vi "Dashboard Main.vi"() -> ()   [LabVIEW 2017]
uses:
  <vilib>/Rock Robotics/Network Tables/NT Read Numeric Array.vi
  <vilib>/Rock Robotics/Network Tables/NT Read Number.vi
  <vilib>/Rock Robotics/Network Tables/NT Write Numeric Array.vi
panel:
  out "Camera Info":cluster{"Mbps LED":bool, "Mbps":dbl, "fps":dbl} {"fps" format="%#.1g"; "Mbps" format="%#.1g"}
  in  "Camera Settings":T1={"Frame Rate"=30, "Compression"=30, "Size"=1, "DB Camera Config"=FALSE} {"Frame Rate" scale=1.0..30.0; "Compression" scale=100.0..-1.0; "Size" items=["640x480", "320x240", "160x120"]}
  in  "TCP":refnum<k5>
  out "Robot IP":string
  in  "Dashboard Tab":T2(tab)
  in  "Select Auto":string(combo)="Select Autonomous ..."
  out "NT Connection":bool
  out "MotorChart R":cluster{"Numeric":dbl, "Numeric":dbl}(graph)
  out "MotorChart L":cluster{"Numeric":dbl, "Numeric":dbl}(graph)
  out "MotorSliders R":cluster{"MotorSlide1":dbl, "MotorSlide2":dbl} {"MotorSlide2" scale=-1.0..1.0 scale format="%#_2e"; "MotorSlide1" scale=-1.0..1.0 scale format="%#_2e"}
  out "MotorSliders L":cluster{"MotorSlide1":dbl, "MotorSlide2":dbl} {"MotorSlide2" scale=-1.0..1.0 scale format="%#_2e"; "MotorSlide1" scale=-1.0..1.0 scale format="%#_2e"}
  out "JS1 Z":dbl(slide) scale=-1.0..1.0 scale format="%#_2e"
  out "JS1 Graph":cluster{"X":dbl, "Y":dbl}[](graph)
  out "JS1 Buttons":T3
  out "JS2 Z":dbl(slide) scale=-1.0..1.0 scale format="%#_2e"
  out "JS2 Graph":cluster{"X":dbl, "Y":dbl}[](graph)
  out "JS2 Buttons":T3
  out "Mode":T4(ring)=enum."Auto Disabled"
  out "Encoder Graph":dbl[][](graph)
  out "JS1 Graph 2":cluster{"X":dbl, "Y":dbl}[](graph)
  out "JS1 Z 2":dbl(slide) scale=-1.0..1.0 scale format="%#_2e"
  out "Waveform Graph":dbl[][](graph)
  in  "P-Value":dbl(slide) scale=-2.0..2.0
  in  "I-Value":dbl(slide) scale=-2.0..2.0
  in  "D-Value":dbl(slide) scale=-2.0..2.0
  in  "H-Lower":dbl(slide) scale=0.0..179.0
  in  "V-Lower":dbl(slide) scale=0.0..255.0
  in  "S-Lower":dbl(slide) scale=0.0..255.0
  in  "S-Higher":dbl(slide) scale=0.0..255.0
  in  "V-Higher":dbl(slide) scale=0.0..255.0
  in  "H-Upper":dbl(slide) scale=0.0..179.0
  out "Tree":string(tree)
  out "Camera Image":T5(plugin-control)
  out "Background":bool
  in  "Camera Name":string(combo)="No Camera Selection"
  # "HW"
  # "Joysticks"
  # "Drive Motors"
  # "Front"
  # "Right"
  # "Left"
  # "Back"
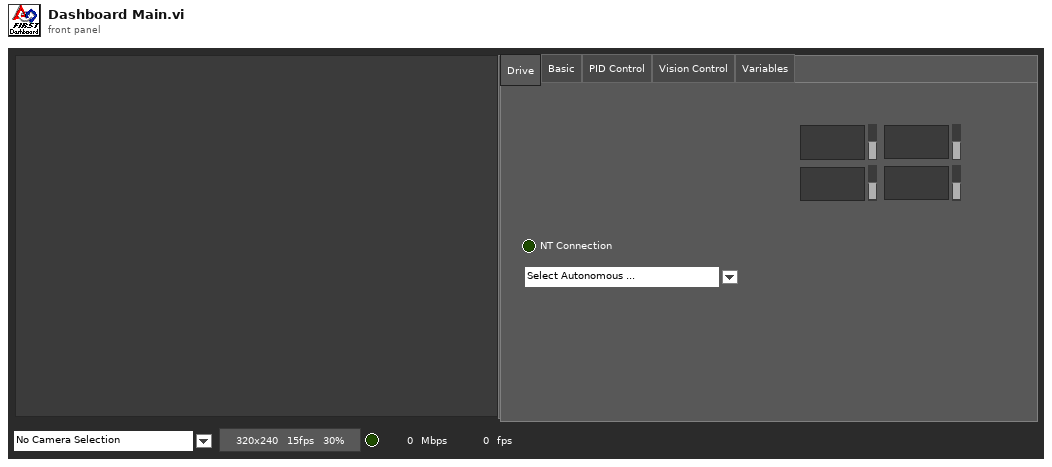
[diagram p1: front panel]
types:
  T1 = cluster{"Frame Rate":i32, "Compression":i32, "Size":u16, "DB Camera Config":bool}
  T2 = enum32{"Drive", "Basic", "PID Control", "Vision Control", "Variables"}
  T3 = cluster{bool, bool, bool, bool, bool, bool, bool, bool, bool, bool, bool, bool}
  T4 = enum8{"Tele-Op Disabled", "Tele-Op Enabled", "Auto Disabled", "Auto Enabled", "Test Disabled", "Test Enabled", "Disconnected", "No Code", "E-Stop"}
  T5 = typedef "IMAQ Image.ctl" = refnum<image>
  T6 = cluster{"Save Path":path, "Interval (s)":dbl, "Keep":i32}
  T7 = typedef "Image Type" = u32
  T8 = cluster{"Camera Image":refnum<vi>, "Dashboard Tab":refnum<vi>, "Background":refnum<vi>, "Tree":refnum<vi>, "Camera Settings":refnum<vi>, "Camera Name":refnum<vi>, "Camera Info":refnum<vi>}
  T9 = cluster{"Shift":bool, "Ctrl":bool, "Alt":bool, "Cmd":bool, "Opt":bool}
  T10 = cluster{"Error Strings":string, "Disable Counts":cluster{u16, u16}, "Rail Faults":cluster{u16, u16, u16}, "Robot IP":string, "DB Mode":u8, "Event Info":cluster{"Name":string, "Type":u8, "Number":u16, "Replay":u8}}
  T11 = cluster{"Storage":cluster{"Disk Free":u64, "RAM Block":u32, "RAM free":u32}, "CPU Utilization":cluster{"CPU % ISR":sgl, "CPU % Time Crit":sgl, "CPU % Timed Str":sgl, "CPU % High":sgl, "CPU % Above":sgl, "CPU % Normal":sgl, "CPU % Low":sgl}, "CAN":cluster{"% Bus Utilization":sgl, "Bus Off Cnt":u32, "TX_FIFO Full Cnt":u32, "Receive Error Cnt":u8, "Transmit Error Cnt":u8}, "HID":cluster{"HID Outputs":u32, "Rumble Low":u16, "Rumble High":u16}[]}
  T12 = cluster{"Status bits":cluster{"Test Mode":bool, "Autonomous":bool, "Enabled":bool, "Code Start":bool, "Brownout":bool, "Reserved 2":bool, "Reserved 3":bool, "E-Stop":bool}, "Code Trace":cluster{"Disabled":bool, "TeleOp":bool, "Auto":bool, "Test":bool}, "Controller Type":enum16{"unknown", "cRIO", "roboRio"}, "Code?":enum16{"unknown", "noCode", "code"}, "Battery V":dbl}
  T13 = cluster{"Control Bits":cluster{"TestMode":bool, "Autonomous":bool, "Enabled":bool, "FMS Present":bool, bool, bool, bool, "E-Stop":bool}, "Team Station ":u8, "Countdown":sgl, "Joystick Values":cluster{"Axes":dbl[], "Buttons":bool[], "POVs":i16[]}[]}
  T14 = cluster{"Axes":dbl[], "Buttons":bool[], "POVs":i16[]}[]
  T15 = cluster{"Axes":dbl[], "Buttons":bool[], "POVs":i16[]}
  T16 = cluster{"Buttons[0]":bool, "Buttons[1]":bool, "Buttons[2]":bool, "Buttons[3]":bool, "Buttons[4]":bool, "Buttons[5]":bool, "Buttons[6]":bool, "Buttons[7]":bool, "Buttons[8]":bool, "Buttons[9]":bool, "Buttons[10]":bool, "Buttons[11]":bool}
  T17 = cluster{"Camera Name":string, "Camera File Name":string, "Saved DB Images Info":cluster{"Save Path":path, "Interval (s)":dbl, "Keep":i32}}
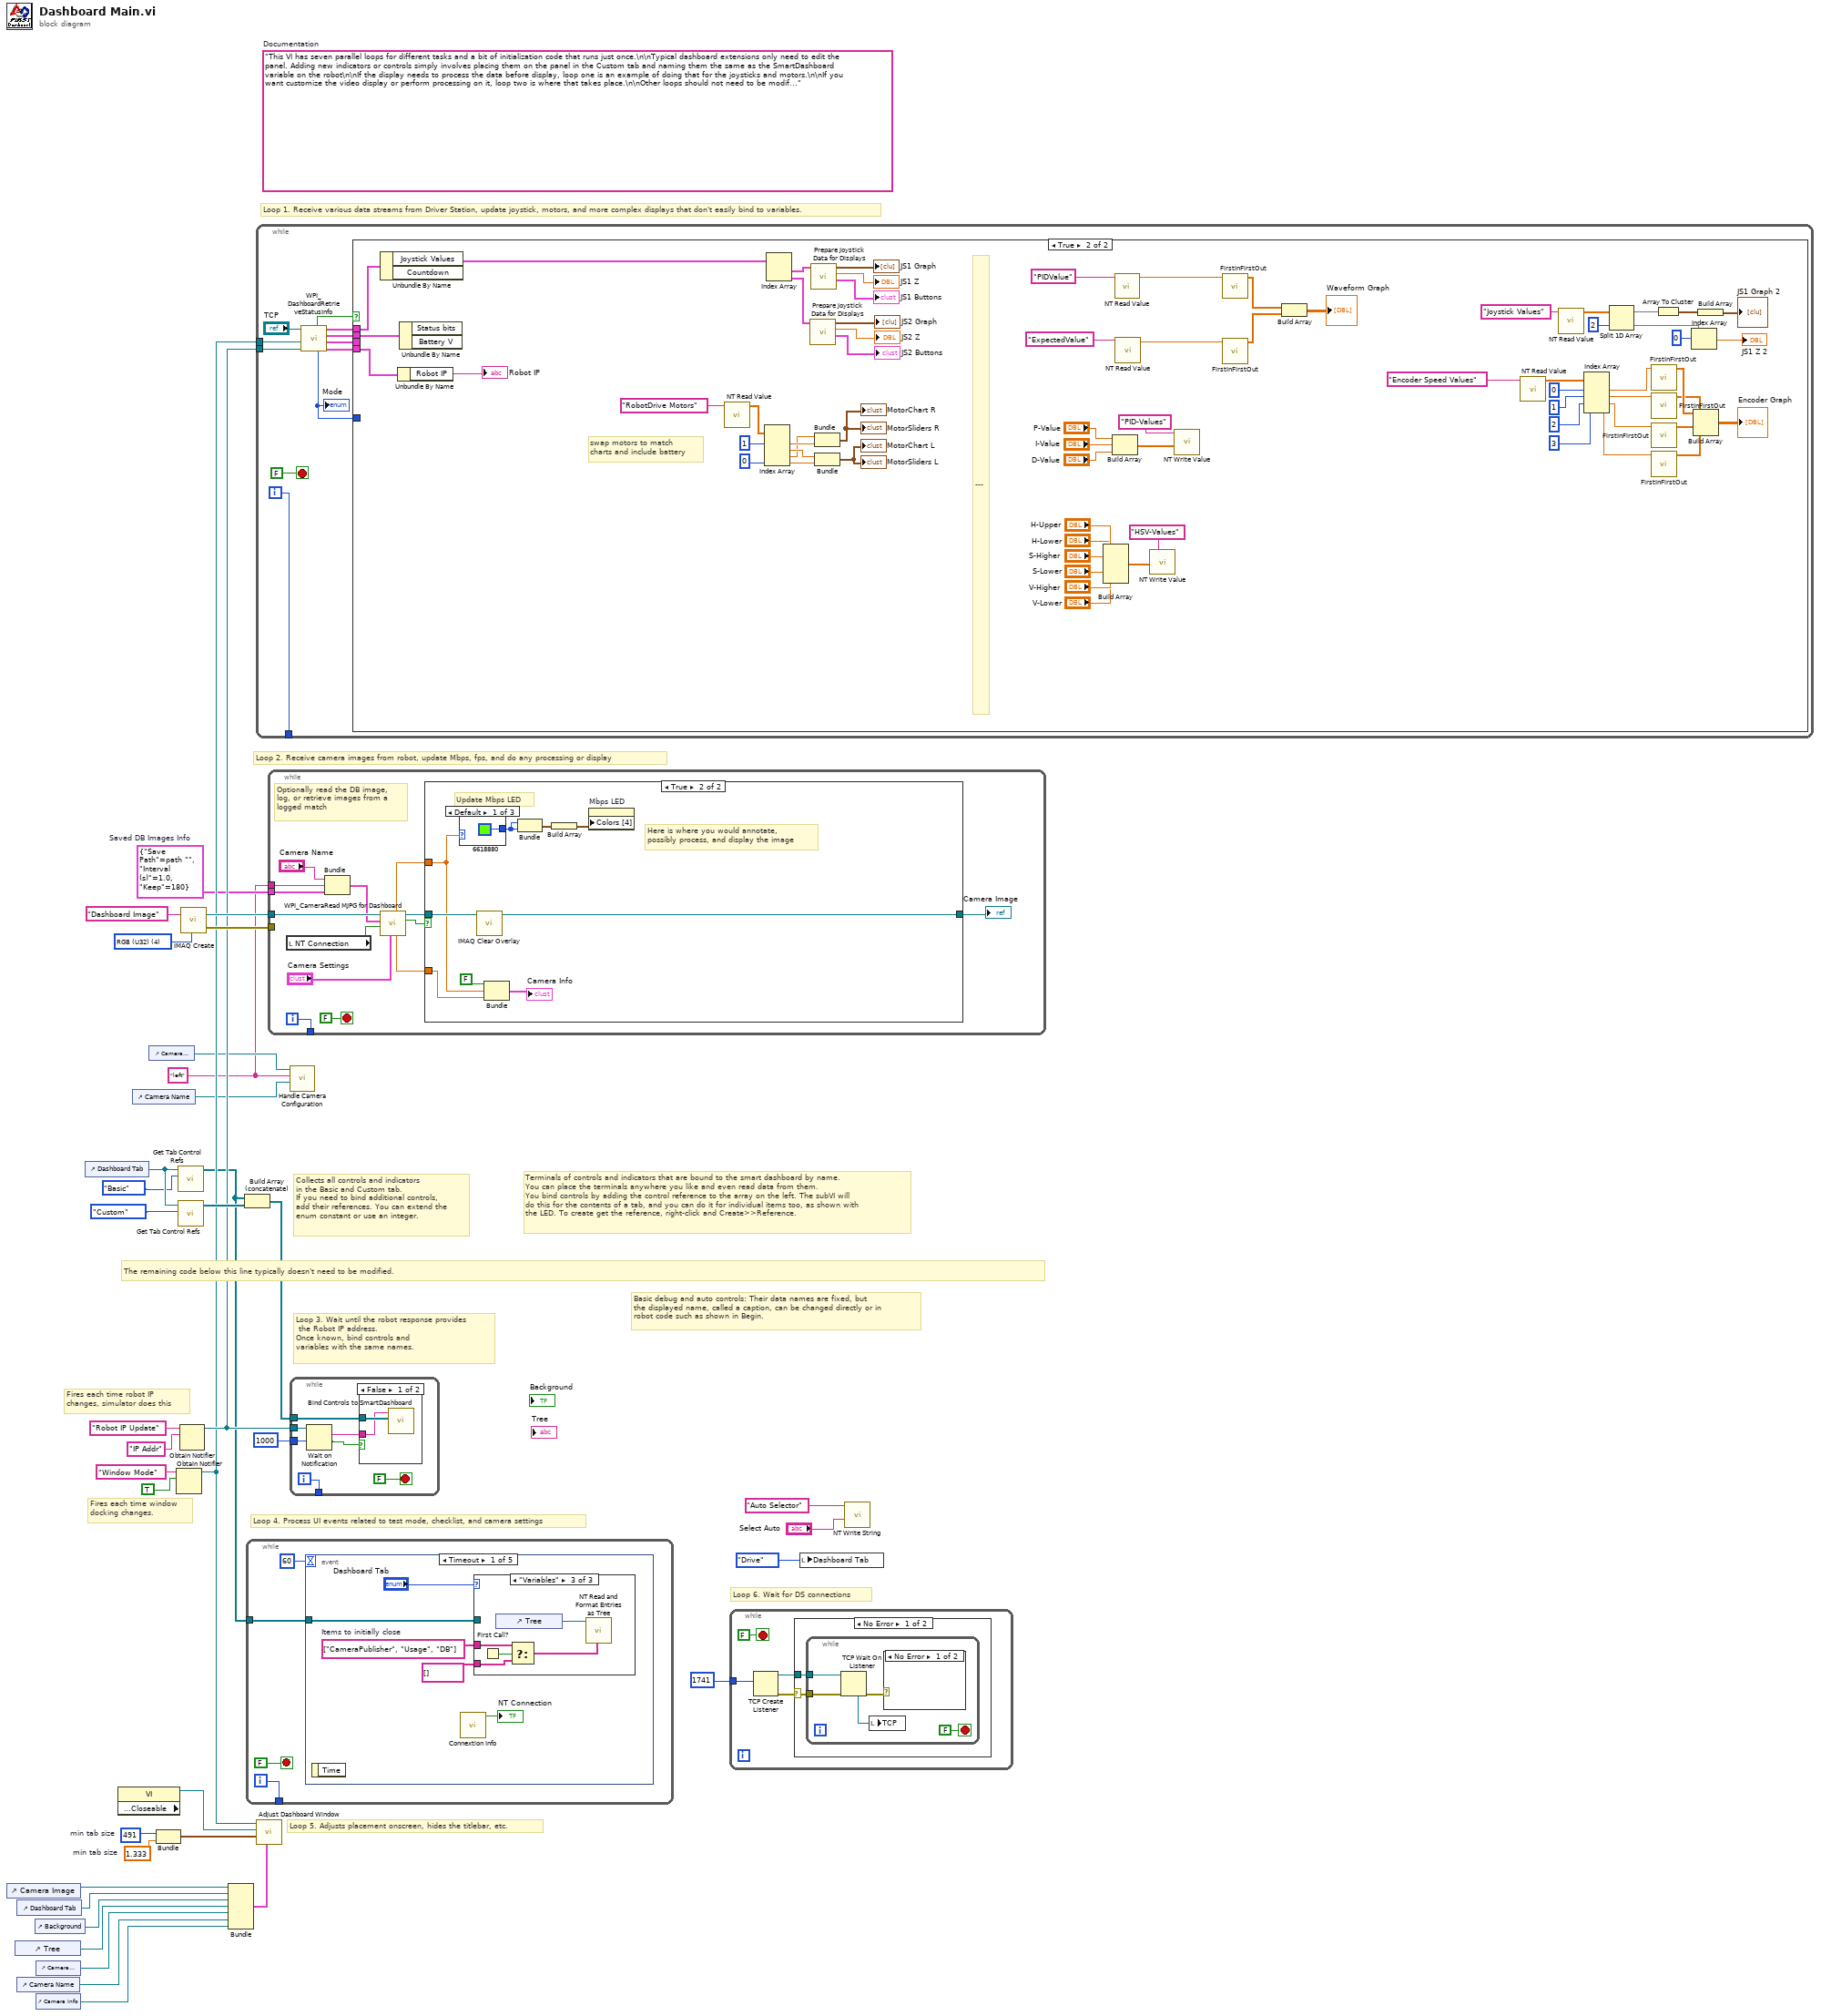
[diagram p0: block diagram]
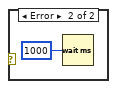
[diagram p2: hidden frame]
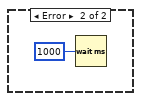
[diagram p3: hidden frame]
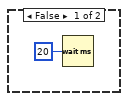
[diagram p4: hidden frame]
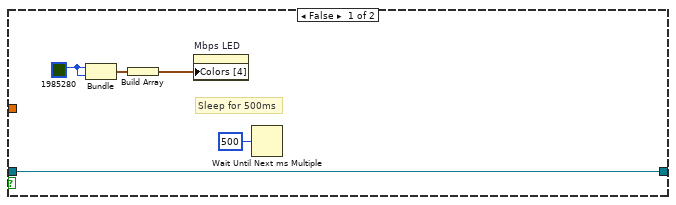
[diagram p6: hidden frame]
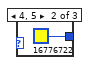
[diagram p7: hidden frame]
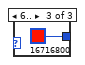
[diagram p8: hidden frame]
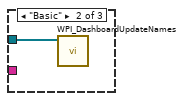
[diagram p10: hidden frame]
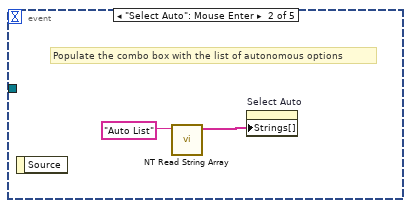
[diagram p11: hidden frame]
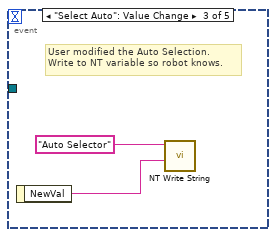
[diagram p12: hidden frame]
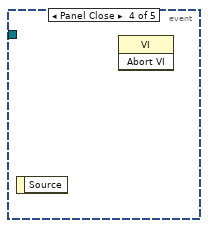
[diagram p13: hidden frame]
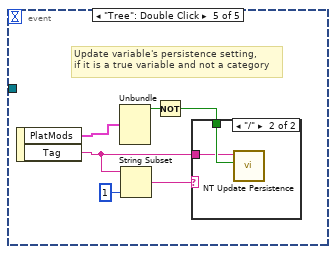
[diagram p14: hidden frame]
diagram:
  w1 = "left" ("Camera File Name")
  w2 = T6 {"Save Path"=path "", "Interval (s)"=1.0, "Keep"=180}  # Saved DB Images Info
  w22 = 491  # min tab size
  w21 = 1.333  # min tab size
  (unwired) "This VI has seven parallel loops for different tasks and a bit of initialization code that runs just once.\n\nTypical dashboard extensions only need to edit the panel. Adding new indicators or controls simply involves placing them on the panel in the Custom tab and naming them the same as the SmartDashboard variable on the robot\n\nIf the display needs to process the data before display, loop one is an example of doing that for the joysticks and motors.\n\nIf you want customize the video display or perform processing on it, loop two is where that takes place.\n\nOther loops should not need to be modified. They are pretty standard, and document the task they perform."  # Documentation
  w37 = T7 4 items=["Grayscale (U8)", "Grayscale (I16)", "Grayscale (SGL)", "Complex (CSG)", "RGB (U32)", "HSL (U32)", "RGB (U64)"] ("Image Type")
  # "Loop 6. Wait for DS connections"
  # "Basic debug and auto controls: Their data names are fixed, but\nthe displayed name, called a caption, can be changed directly or in\nrobot code such as shown in Begin."
  # "Fires each time robot IP\nchanges, simulator does this"
  # "Fires each time window\ndocking changes."
  # "Collects all controls and indicators\nin the Basic and Custom tab.\nIf you need to bind additional controls,\nadd their references. You can extend the\nenum constant or use an integer."
  # "The remaining code below this line typically doesn't need to be modified."
  # "Loop 4. Process UI events related to test mode, checklist, and camera settings"
  # "Terminals of controls and indicators that are bound to the smart dashboard by name.\nYou can place the terminals anywhere you like and even read data from them.\nYou bind controls by adding the control reference to the array on the left. The subVI will\ndo this for the contents of a tab, and you can do it for individual items too, as shown with\nthe LED. To create get the reference, right-click and Create>>Reference."
  # "Loop 3. Wait until the robot response provides\n the Robot IP address.\nOnce known, bind controls and\nvariables with the same names."
  # "Loop 5. Adjusts placement onscreen, hides the titlebar, etc."
  # "Loop 1. Receive various data streams from Driver Station, update joystick, motors, and more complex displays that don't easily bind to variables."
  # "Loop 2. Receive camera images from robot, update Mbps, fps, and do any processing or display"
  n1 = control-ref of="Camera Image"() -> (w24:refnum<vi>)
  n2 = control-ref of="Tree"() -> (w8:refnum<vi>)
  n3 = control-ref of="Dashboard Tab"() -> (w23:refnum<vi>)
  n4 = control-ref of="Camera Name"() -> (w6:refnum<vi>)
  n5 = control-ref of="Background"() -> (w19:refnum<vi>)
  n6 = control-ref of="Camera Settings"() -> (w7:refnum<vi>)
  n7 = control-ref of="Camera Info"() -> (w5:refnum<vi>)
  n8 = control-ref of="Dashboard Tab"() -> (w27:refnum<vi>)
  n9 = property class="VI" props=["Front Panel.Closeable"]() -> (reference out=w28:refnum<vi>)  [unwired: 2 in, 2 out]
  n10 = control-ref of="Camera Name"() -> (w12:refnum<vi>)
  n11 = control-ref of="Camera Settings"() -> (w13:refnum<vi>)
  n12 = Bundle("min tab size"=w22, "min tab size"=w21) -> (w20:cluster{"min tab size":i32, "min tab size":dbl})  [unwired: 1 in]
  n13 = Obtain Notifier(name (unnamed)="Window Mode", notification data type=TRUE) -> (notifier out=w16:refnum<notifier>)  [unwired: 2 in, 2 out]
  n14 = call <vilib>:"Get Tab Control Refs.vi"("Page Index"=enum32{"Drive", "Basic", "Custom", "Variables"}."Basic" ("Dashboard Tab"), "TabControl in"=w27) -> ("ControlsOnPage"=w11:refnum<vi>[])  [unwired: 9 in]
  n15 = call <vilib>:"Get Tab Control Refs.vi"("Page Index"=enum32{"Drive", "Basic", "Custom", "Variables"}."Custom" ("Dashboard Tab"), "TabControl in"=w27) -> ("ControlsOnPage"=w26:refnum<vi>[])  [unwired: 9 in]
  n16 = Obtain Notifier(name (unnamed)="Robot IP Update", notification data type="IP Addr" ("name (unnamed)")) -> (notifier out=w17:refnum<notifier>)  [unwired: 2 in, 2 out]
  n17 = call "IMAQ Create"("Image Name"="Dashboard Image", "Image Type"=w37) -> ("New Image"=w35:T5, "error out"=w34:errorcluster)  [unwired: 2 in, 1 out]
  n18 = Bundle("Camera Image"=w24, "Dashboard Tab"=w23, "Background"=w19, "Tree"=w8, "Camera Settings"=w7, "Camera Name"=w6, "Camera Info"=w5) -> (w18:T8)  [unwired: 1 in]
  n19 = Build Array (concatenate)(w11, w26) -> (w25:refnum<vi>[])
  n20 = while {
    tunnel: [w39] -> _
    tunnel: w11 -> [w38]
    i -> [w39]
    stop <- FALSE stop-if-true
    n21 = event shown="[0] Timeout" {
      selector: _ -> [_ _ _ _ _]
      dyn-events: _ -> [_ _ _ _ _]
      timeout: u32 60 ("milliseconds to wait") -> [_ _ _ _ _]
      tunnel: w38 -> [w44 _ _ _ _]
      event Timeout {
        w43 = string[] ["CameraPublisher", "Usage", "DB"]  # Items to initially close
        n22 = event-data() -> ()  [unwired: 1 in, 1 out]
        n23 = call <vilib>:"Connextion Info.vi"() -> ("Connected"=→"NT Connection":bool)  [unwired: 10 in, 1 out]
        n24 = case shown="\"Variables\"" "Dashboard Tab" {
          tunnel: w44 -> [_ w47 _]
          tunnel: w43 -> [_ _ w50]
          tunnel: string[] [] -> [_ _ w49]
          frame "PID Control", Default {
          }
          frame "Basic" {
            n25 = call <vilib>:"WPI_DashboardUpdateNames.vi"("Controls on Tab"=w47) -> ()  [unwired: 11 in]
          }
          frame "Variables" {
            n26 = First Call?() -> (First Call?: T/F=w51:bool)
            n27 = control-ref of="Tree"() -> (w52:refnum<vi>)
            n28 = Select(t=w50, s=w51, f=w49) -> (s? t:f=w48:string[])
            n29 = call <vilib>:"NT Read and Format Entries as Tree.vi"("Tags to  Close"=w48, "Tree Refnum"=w52) -> ()  [unwired: 8 in, 2 out]
          }
        }
      }
      event "Select Auto": Mouse Enter {
        # "Populate the combo box with the list of autonomous options"
        n30 = event-data() -> ()  [unwired: 1 in, 1 out]
        n31 = call <vilib>:"NT Read String Array.vi"("Name"="Auto List") -> ("String Array"=w53:string[])  [unwired: 9 in, 1 out]
        n32 = property on="Select Auto" class="CmbBox"("Strings[]"=w53) -> ()  [unwired: 2 in, 2 out]
      }
      event "Select Auto": Value Change {
        # "User modified the Auto Selection.\nWrite to NT variable so robot knows."
        n33 = event-data() -> ("NewVal"=w55:string)  [unwired: 1 in]
        n34 = call <vilib>:"NT Write String.vi"("String"=w55, "Name"="Auto Selector") -> ()  [unwired: 9 in, 1 out]
      }
      event Panel Close {
        n35 = event-data() -> ()  [unwired: 1 in, 1 out]
        n36 = invoke class="VI" method="Abort VI"() -> ()  [unwired: 3 in, 3 out]
      }
      event "Tree": Double Click {
        # "Update variable's persistence setting,\nif it is a true variable and not a category"
        n37 = event-data() -> ("PlatMods"=w58:T9, "Tag"=w57:string)  [unwired: 1 in]
        n38 = Unbundle(w58) -> ("Shift"=w62:bool)  [unwired: 4 out]
        n39 = String Subset(string=w57, length (rest)=1 ("length (rest)")) -> (substring=w59:string)  [unwired: 1 in]
        n40 = Not(x=w62) -> (.not. x?=w61:bool)
        n41 = case shown="\"/\"" w59 {
          tunnel: w61 -> [_ w64]
          tunnel: w57 -> [_ w63]
          frame Default {
          }
          frame "/" {
            n42 = call <vilib>:"NT Update Persistence.vi"("Persistence"=w64, "Name"=w63) -> ()  [unwired: 9 in, 1 out]
          }
        }
      }
    }
  }
  n43 = while {
    tunnel: [w74] -> _
    tunnel: w17 -> [w68]
    tunnel: w16 -> [w65]
    i -> [w74]
    stop <- FALSE stop-if-true
    n44 = call <vilib>:"WPI_DashboardRetrieveStatusInfo.vi"("Binding Refnum"=w68, "Window Mode Notifier"=w65, "TCP Cnx"="TCP") -> ("Power and Errors"=w69:T10, "Robot Metrics"=w72:T11, "Status Info"=w73:T12, "Control Info"=w70:T13, "Robot Mode"=w67:T4, "Process?"=w71:bool)  [unwired: 3 in]
    "Mode" <- w67
    n45 = case shown="True" w71 {
      tunnel: w73 -> [_ w143]
      tunnel: w72 -> [_ _]
      tunnel: w70 -> [_ w142]
      tunnel: w69 -> [_ w141]
      tunnel: w67 -> [_ _]
      frame False {
        n46 = Wait (ms)(milliseconds to wait=u32 20) -> ()  [unwired: 1 out]
      }
      frame True {
        # "---"
        # "swap motors to match\ncharts and include battery"
        n47 = Unbundle By Name(w142) -> ("Joystick Values"=w132:T14)  [unwired: 1 out]
        n48 = Unbundle By Name(w141) -> ("Robot IP"=→"Robot IP":string)
        n49 = Unbundle By Name(w143) -> ()  [unwired: 2 out]
        n50 = call-poly <vilib>:"NT Read Value.vi"("Name"="RobotDrive Motors") -> ("Numeric Array"=w122:dbl[])  [unwired: 9 in, 1 out]
        n51 = Index Array(array=w122, index #1=1, index #4=0) -> (element #1=w136:dbl, element #2=w137:dbl, element #3=w135:dbl, element #4=w140:dbl)  [unwired: 2 in]
        n52 = Index Array(array=w132) -> (element #1=w131:T15, element #2=w127:T15)  [unwired: 2 in]
        n53 = call "Prepare Joystick Data for Displays.vi"("Joystick Values"=w127) -> ("Buttons"=→"JS2 Buttons":T16, "Z Axis"=→"JS2 Z":dbl, "Cartesian Data"=→"JS2 Graph":cluster{"X axis":dbl, "X axis":dbl}[])  [unwired: 8 in]
        n54 = call "Prepare Joystick Data for Displays.vi"("Joystick Values"=w131) -> ("Buttons"=→"JS1 Buttons":T16, "Z Axis"=→"JS1 Z":dbl, "Cartesian Data"=→"JS1 Graph":cluster{"X axis":dbl, "X axis":dbl}[])  [unwired: 8 in]
        n55 = Bundle("Numeric"=w135, "Numeric"=w136) -> (→"MotorChart R" →"MotorSliders R":cluster{"Numeric":dbl, "Numeric":dbl})  [unwired: 1 in]
        n56 = Bundle("Numeric"=w137, "Numeric"=w140) -> (→"MotorChart L" →"MotorSliders L":cluster{"Numeric":dbl, "Numeric":dbl})  [unwired: 1 in]
        n57 = Build Array("H-Upper", "H-Lower", "S-Higher", "S-Lower", "V-Higher", "V-Lower") -> (w77:dbl[])
        n58 = Build Array("P-Value", "I-Value", "D-Value") -> (w110:dbl[])
        n59 = call-poly <vilib>:"NT Read Value.vi"("Name"="PIDValue") -> ("Numeric"=w120:dbl)  [unwired: 9 in, 1 out]
        n60 = call-poly <vilib>:"NT Read Value.vi"("Name"="ExpectedValue") -> ("Numeric"=w116:dbl)  [unwired: 9 in, 1 out]
        n61 = call-poly <vilib>:"NT Write Value.vi"("Numeric Array"=w77, "Name"="HSV-Values") -> ()  [unwired: 9 in, 1 out]
        n62 = call-poly <vilib>:"NT Write Value.vi"("Numeric Array"=w110, "Name"="PID-Values") -> ()  [unwired: 9 in, 1 out]
        n63 = call "FirstInFirstOut.vi"("Input"=w120) -> ("Output"=w114:dbl[])  [unwired: 10 in]
        n64 = call "FirstInFirstOut.vi"("Input"=w116) -> ("Output"=w115:dbl[])  [unwired: 10 in]
        n65 = Build Array(w114, w115) -> (→"Waveform Graph":dbl[][])
        n66 = call-poly <vilib>:"NT Read Value.vi"("Name"="Encoder Speed Values") -> ("Numeric Array"=w98:dbl[])  [unwired: 9 in, 1 out]
        n67 = call-poly <vilib>:"NT Read Value.vi"("Name"="Joystick Values") -> ("Numeric Array"=w108:dbl[])  [unwired: 9 in, 1 out]
        n68 = Index Array(array=w98, index #1=0, index #2=1, index #3=2, index #4=3) -> (element #1=w93:dbl, element #2=w92:dbl, element #3=w91:dbl, element #4=w90:dbl)
        n69 = Split 1D Array(array=w108, index=2) -> (first subarray=w104:dbl[], second subarray=w106:dbl[])
        n70 = call "FirstInFirstOut.vi"("Input"=w93) -> ("Output"=w89:dbl[])  [unwired: 10 in]
        n71 = call "FirstInFirstOut.vi"("Input"=w92) -> ("Output"=w88:dbl[])  [unwired: 10 in]
        n72 = call "FirstInFirstOut.vi"("Input"=w91) -> ("Output"=w87:dbl[])  [unwired: 10 in]
        n73 = call "FirstInFirstOut.vi"("Input"=w90) -> ("Output"=w86:dbl[])  [unwired: 10 in]
        n74 = Array To Cluster(array=w104) -> (cluster=w103:cluster{"[0]":dbl, "[1]":dbl})
        n75 = Index Array(array=w106, index=0) -> (element=→"JS1 Z 2":dbl)
        n76 = Build Array(w89, w88, w87, w86) -> (→"Encoder Graph":dbl[][])
        n77 = Build Array(w103) -> (→"JS1 Graph 2":cluster{"[0]":dbl, "[1]":dbl}[])
      }
    }
  }
  n78 = call "Adjust Dashboard Window.vi"("Sizing Refnums"=w18, "Size Constraints"=w20, "VI"=w28, "WIn Mode"=w16) -> ()  [unwired: 8 in]
  n79 = while {
    tunnel: w35 -> [w155]
    tunnel: w34 -> [_]
    tunnel: [w156] -> _
    tunnel: w2 -> [w147]
    tunnel: w1 -> [w144]
    i -> [w156]
    stop <- FALSE stop-if-true
    # "Optionally read the DB image,\nlog, or retrieve images from a\nlogged match"
    n80 = local read "NT Connection"() -> (w148:bool)
    n81 = Bundle("Camera Name"="Camera Name", "Camera File Name"=w144, "Saved DB Images Info"=w147) -> (w146:T17)  [unwired: 1 in]
    n82 = call <vilib>:"WPI_CameraRead MJPG for Dashboard.vi"("Camera Settings"="Camera Settings", "NT Connection"=w148, "Capture Info"=w146, "Refnum in"=w155) -> ("Active"=w153:bool, "Refnum out"=w154:T5, "FPS"=w152:dbl, "Bandwidth (Mbps)"=w151:dbl)  [unwired: 4 in]
    n83 = case shown="True" w153 {
      tunnel: w154 -> [w158 w169]
      tunnel: w151 -> [_ w166]
      tunnel: w152 -> [_ w167]
      tunnel: [w158 w163] -> w149
      frame False {
        w160 = u32 1985280 ("Color Box")
        # "Sleep for 500ms"
        n84 = Bundle("Color Box"=w160, "Color Box"=w160) -> (w161:cluster{"Color Box":u32, "Color Box":u32})  [unwired: 1 out]
        n85 = Build Array(w161) -> (w159:cluster{"Color Box":u32, "Color Box":u32}[])
        n86 = property on="Mbps LED" class="Bool (strict)"("Colors [4]"=w159) -> ()  [unwired: 2 in, 2 out]
        n87 = Wait Until Next ms Multiple(millisecond multiple=u32 500) -> ()  [unwired: 1 out]
      }
      frame True {
        # "Here is where you would annotate,\npossibly process, and display the image"
        # "Update Mbps LED"
        n88 = case shown="Default" w166 {
          tunnel: [u32 6618880 ("Color Box") u32 16776722 ("Color Box") u32 16716800 ("Color Box")] -> w170
          frame Default {
          }
          frame 4, 5 {
          }
          frame 6.. {
          }
        }
        n89 = call "IMAQ Clear Overlay"("Image"=w169) -> ("Image Out"=w163:T5)  [unwired: 2 in, 8 out]
        n90 = Bundle(FALSE, "Bandwidth (Mbps)"=w166, "FPS"=w167) -> (→"Camera Info":cluster{bool, "Bandwidth (Mbps)":dbl, "FPS":dbl})  [unwired: 1 in]
        n91 = Bundle("Color Box"=w170, "Color Box"=w170) -> (w171:cluster{"Color Box":u32, "Color Box":u32})  [unwired: 1 out]
        n92 = Build Array(w171) -> (w168:cluster{"Color Box":u32, "Color Box":u32}[])
        n93 = property on="Mbps LED" class="Bool (strict)"("Colors [4]"=w168) -> ()  [unwired: 2 in, 2 out]
      }
    }
    "Camera Image" <- w149
  }
  n94 = call "Handle Camera Configuration.vi"("CameraNameRef"=w12, "Camera File Name"=w1, "ClusterRef"=w13) -> ()  [unwired: 9 in]
  n95 = while {
    tunnel: w25 -> [w181]
    tunnel: w17 -> [w179]
    tunnel: [w177] -> _
    tunnel: u32 1000 ("milliseconds to wait") -> [w176]
    i -> [w177]
    stop <- FALSE stop-if-true
    n96 = Wait on Notification(notifier=w179, timeout in ms (-1)=w176) -> (notification=w178:string, timed out?=w175:bool)  [unwired: 2 in, 2 out]
    n97 = case shown="False" w175 {
      tunnel: w181 -> [w183 _]
      tunnel: w178 -> [w182 _]
      frame False {
        n98 = call <vilib>:"Bind Controls to SmartDashboard.vi"("Bound Control Refs"=w183, "Server IP Address"=w182) -> ()  [unwired: 10 in]
      }
      frame True {
      }
    }
  }
  n99 = while {
    tunnel: u16 1741 ("timeout ms (25000)") -> [w185]
    stop <- FALSE stop-if-true
    n100 = TCP Create Listener(10:w185) -> (0:w184:errorcluster, 3:w186:refnum<k5>)  [unwired: 4 in, 1 out]
    n101 = case shown="No Error" w184 {
      selector: w184 -> [w188 _]
      tunnel: w186 -> [w189 _]
      frame No Error {
        n102 = while {
          tunnel: w189 -> [w192]
          tunnel: w188 -> [w191]
          stop <- FALSE stop-if-true
          n103 = TCP Wait On Listener(8:w191, 11:w192) -> (0:w193:errorcluster, 4:w194:refnum<k5>)  [unwired: 2 in, 3 out]
          n104 = local write "TCP"(w194) -> ()
          n105 = case shown="No Error" w193 {
            frame No Error {
            }
            frame Error {
              n106 = Wait (ms)(milliseconds to wait=u32 1000) -> ()  [unwired: 1 out]
            }
          }
        }
      }
      frame Error {
        n107 = Wait (ms)(milliseconds to wait=u32 1000) -> ()  [unwired: 1 out]
      }
    }
  }
  n108 = local write "Dashboard Tab"(T2."Drive" ("Dashboard Tab")) -> ()
  n109 = call <vilib>:"NT Write String.vi"("String"="Select Auto", "Name"="Auto Selector") -> ()  [unwired: 9 in, 1 out]
